vi "Lab Panel V4.90.vi"() -> ()   [LabVIEW 2013] (continued)
                    n2521 = local read "SIG LAB02-2"() -> (w4767:T2)
                    n2522 = local read "RESULT LAB02-2"() -> (w4754:bool)
                    n2523 = Bundle("FAIL LAB02-2"=w4757, "SIG LAB02-2"=w4767, "TEMP START LAB02-2"=w4766, "DISP LAB02-2"=w4763, "SET LAB02-2"=w4762, "TDMS LAB02-2"=w4765) -> (w4752:T35)  [unwired: 1 in]
                    n2524 = call "sub vi - cycle&temp fail v7.vi"("Amps Lo?"=w4764, "Input Cluster"=w4752, "SELECT"=w4761, "Amps Hi?"=w4760, "Result In"=w4754) -> ("(FAIL) out"=w4756:cluster{"FAIL LO":dbl, "FAIL HI":dbl}, "(DISP) out"=w4759:T4, "T-RISE"=w4753:cluster{"T-RISE (L)":dbl, "T-RISE (N)":dbl}, "Result Out"=w4755:bool, "file error"=w4758:errorcluster)  [unwired: 10 in]
                    n2525 = local write "TEMP RISE LAB02-2"(w4753) -> ()
                    n2526 = local write "FAIL LAB02-2"(w4756) -> ()
                    n2527 = local write "DISP LAB02-2"(w4759) -> ()
                    n2528 = local write "RESULT LAB02-2"(w4755) -> ()
                    n2529 = local write "data file error"(w4758) -> ()
                  }
                }
              }
              frame #4 {
                # "LAB03-1"
                n2530 = case shown="True" w4769 {
                  tunnel: w4771 -> [_ w4784]
                  tunnel: w4768 -> [_ w4781]
                  tunnel: w4770 -> [_ w4780]
                  frame False {
                  }
                  frame True {
                    n2531 = local read "TEMP START LAB03-1"() -> (w4786:cluster{"TL":dbl, "TN":dbl})
                    n2532 = local read "FAIL LAB03-1"() -> (w4777:cluster{"LO":dbl, "HI":dbl})
                    n2533 = local read "TDMS LAB03-1"() -> (w4785:refnum<k34>)
                    n2534 = local read "SET LAB03-1"() -> (w4782:T5)
                    n2535 = local read "DISP LAB03-1"() -> (w4783:T4)
                    n2536 = local read "SIG LAB03-1"() -> (w4787:T2)
                    n2537 = local read "RESULT LAB03-1"() -> (w4774:bool)
                    n2538 = Bundle("FAIL LAB03-1"=w4777, "SIG LAB03-1"=w4787, "TEMP START LAB03-1"=w4786, "DISP LAB03-1"=w4783, "SET LAB03-1"=w4782, "TDMS LAB03-1"=w4785) -> (w4772:T36)  [unwired: 1 in]
                    n2539 = call "sub vi - cycle&temp fail v7.vi"("Amps Lo?"=w4784, "Input Cluster"=w4772, "SELECT"=w4781, "Amps Hi?"=w4780, "Result In"=w4774) -> ("(FAIL) out"=w4776:cluster{"FAIL LO":dbl, "FAIL HI":dbl}, "(DISP) out"=w4779:T4, "T-RISE"=w4773:cluster{"T-RISE (L)":dbl, "T-RISE (N)":dbl}, "Result Out"=w4775:bool, "file error"=w4778:errorcluster)  [unwired: 10 in]
                    n2540 = local write "TEMP RISE LAB03-1"(w4773) -> ()
                    n2541 = local write "FAIL LAB03-1"(w4776) -> ()
                    n2542 = local write "DISP LAB03-1"(w4779) -> ()
                    n2543 = local write "RESULT LAB03-1"(w4775) -> ()
                    n2544 = local write "data file error"(w4778) -> ()
                  }
                }
              }
              frame #5 {
                # "LAB03-2"
                n2545 = case shown="True" w4789 {
                  tunnel: w4791 -> [_ w4804]
                  tunnel: w4788 -> [_ w4801]
                  tunnel: w4790 -> [_ w4800]
                  frame False {
                  }
                  frame True {
                    n2546 = local read "TEMP START LAB03-2"() -> (w4806:cluster{"TL":dbl, "TN":dbl})
                    n2547 = local read "FAIL LAB03-2"() -> (w4797:cluster{"LO":dbl, "HI":dbl})
                    n2548 = local read "TDMS LAB03-2"() -> (w4805:refnum<k34>)
                    n2549 = local read "SET LAB03-2"() -> (w4802:T5)
                    n2550 = local read "DISP LAB03-2"() -> (w4803:T4)
                    n2551 = local read "RESULT LAB03-2"() -> (w4794:bool)
                    n2552 = local read "SIG LAB03-2"() -> (w4807:T2)
                    n2553 = Bundle("FAIL LAB03-2"=w4797, "SIG LAB03-2"=w4807, "TEMP START LAB03-2"=w4806, "DISP LAB03-2"=w4803, "SET LAB03-2"=w4802, "TDMS LAB03-2"=w4805) -> (w4792:T37)  [unwired: 1 in]
                    n2554 = call "sub vi - cycle&temp fail v7.vi"("Amps Lo?"=w4804, "Input Cluster"=w4792, "SELECT"=w4801, "Amps Hi?"=w4800, "Result In"=w4794) -> ("(FAIL) out"=w4796:cluster{"FAIL LO":dbl, "FAIL HI":dbl}, "(DISP) out"=w4799:T4, "T-RISE"=w4793:cluster{"T-RISE (L)":dbl, "T-RISE (N)":dbl}, "Result Out"=w4795:bool, "file error"=w4798:errorcluster)  [unwired: 10 in]
                    n2555 = local write "FAIL LAB03-2"(w4796) -> ()
                    n2556 = local write "TEMP RISE LAB03-2"(w4793) -> ()
                    n2557 = local write "DISP LAB03-2"(w4799) -> ()
                    n2558 = local write "RESULT LAB03-2"(w4795) -> ()
                    n2559 = local write "data file error"(w4798) -> ()
                  }
                }
              }
              frame #6 {
                # "LAB04-1"
                n2560 = case shown="True" w4809 {
                  tunnel: w4811 -> [_ w4824]
                  tunnel: w4808 -> [_ w4821]
                  tunnel: w4810 -> [_ w4820]
                  frame False {
                  }
                  frame True {
                    n2561 = local read "TEMP START LAB04-1"() -> (w4826:cluster{"TL":dbl, "TN":dbl})
                    n2562 = local read "FAIL LAB04-1"() -> (w4817:cluster{"LO":dbl, "HI":dbl})
                    n2563 = local read "TDMS LAB04-1"() -> (w4825:refnum<k34>)
                    n2564 = local read "SET LAB04-1"() -> (w4822:T5)
                    n2565 = local read "DISP LAB04-1"() -> (w4823:T4)
                    n2566 = local read "SIG LAB04-1"() -> (w4827:T2)
                    n2567 = local read "RESULT LAB04-1"() -> (w4814:bool)
                    n2568 = Bundle("FAIL LAB04-1"=w4817, "SIG LAB04-1"=w4827, "TEMP START LAB04-1"=w4826, "DISP LAB04-1"=w4823, "SET LAB04-1"=w4822, "TDMS LAB04-1"=w4825) -> (w4812:T38)  [unwired: 1 in]
                    n2569 = call "sub vi - cycle&temp fail v7.vi"("Amps Lo?"=w4824, "Input Cluster"=w4812, "SELECT"=w4821, "Amps Hi?"=w4820, "Result In"=w4814) -> ("(FAIL) out"=w4816:cluster{"FAIL LO":dbl, "FAIL HI":dbl}, "(DISP) out"=w4819:T4, "T-RISE"=w4813:cluster{"T-RISE (L)":dbl, "T-RISE (N)":dbl}, "Result Out"=w4815:bool, "file error"=w4818:errorcluster)  [unwired: 10 in]
                    n2570 = local write "TEMP RISE LAB04-1"(w4813) -> ()
                    n2571 = local write "FAIL LAB04-1"(w4816) -> ()
                    n2572 = local write "DISP LAB04-1"(w4819) -> ()
                    n2573 = local write "RESULT LAB04-1"(w4815) -> ()
                    n2574 = local write "data file error"(w4818) -> ()
                  }
                }
              }
              frame #7 {
                # "LAB04-2"
                n2575 = case shown="True" w4829 {
                  tunnel: w4831 -> [_ w4844]
                  tunnel: w4828 -> [_ w4841]
                  tunnel: w4830 -> [_ w4840]
                  frame False {
                  }
                  frame True {
                    n2576 = local read "TEMP START LAB04-2"() -> (w4846:cluster{"TL":dbl, "TN":dbl})
                    n2577 = local read "FAIL LAB04-2"() -> (w4837:cluster{"LO":dbl, "HI":dbl})
                    n2578 = local read "TDMS LAB04-2"() -> (w4845:refnum<k34>)
                    n2579 = local read "SET LAB04-2"() -> (w4842:T5)
                    n2580 = local read "DISP LAB04-2"() -> (w4843:T4)
                    n2581 = local read "SIG LAB04-2"() -> (w4847:T2)
                    n2582 = local read "RESULT LAB04-2"() -> (w4834:bool)
                    n2583 = Bundle("FAIL LAB04-2"=w4837, "SIG LAB04-2"=w4847, "TEMP START LAB04-2"=w4846, "DISP LAB04-2"=w4843, "SET LAB04-2"=w4842, "TDMS LAB04-2"=w4845) -> (w4832:T39)  [unwired: 1 in]
                    n2584 = call "sub vi - cycle&temp fail v7.vi"("Amps Lo?"=w4844, "Input Cluster"=w4832, "SELECT"=w4841, "Amps Hi?"=w4840, "Result In"=w4834) -> ("(FAIL) out"=w4836:cluster{"FAIL LO":dbl, "FAIL HI":dbl}, "(DISP) out"=w4839:T4, "T-RISE"=w4833:cluster{"T-RISE (L)":dbl, "T-RISE (N)":dbl}, "Result Out"=w4835:bool, "file error"=w4838:errorcluster)  [unwired: 10 in]
                    n2585 = local write "TEMP RISE LAB04-2"(w4833) -> ()
                    n2586 = local write "FAIL LAB04-2"(w4836) -> ()
                    n2587 = local write "DISP LAB04-2"(w4839) -> ()
                    n2588 = local write "RESULT LAB04-2"(w4835) -> ()
                    n2589 = local write "data file error"(w4838) -> ()
                  }
                }
              }
              frame #8 {
                # "LAB05-1"
                n2590 = case shown="True" w4849 {
                  tunnel: w4851 -> [_ w4864]
                  tunnel: w4848 -> [_ w4861]
                  tunnel: w4850 -> [_ w4860]
                  frame False {
                  }
                  frame True {
                    n2591 = local read "TEMP START LAB05-1"() -> (w4866:cluster{"TL":dbl, "TN":dbl})
                    n2592 = local read "FAIL LAB05-1"() -> (w4857:cluster{"LO":dbl, "HI":dbl})
                    n2593 = local read "TDMS LAB05-1"() -> (w4865:refnum<k34>)
                    n2594 = local read "SET LAB05-1"() -> (w4862:T5)
                    n2595 = local read "DISP LAB05-1"() -> (w4863:T4)
                    n2596 = local read "SIG LAB05-1"() -> (w4867:T2)
                    n2597 = local read "RESULT LAB05-1"() -> (w4854:bool)
                    n2598 = Bundle("FAIL LAB05-1"=w4857, "SIG LAB05-1"=w4867, "TEMP START LAB05-1"=w4866, "DISP LAB05-1"=w4863, "SET LAB05-1"=w4862, "TDMS LAB05-1"=w4865) -> (w4852:T40)  [unwired: 1 in]
                    n2599 = call "sub vi - cycle&temp fail v7.vi"("Amps Lo?"=w4864, "Input Cluster"=w4852, "SELECT"=w4861, "Amps Hi?"=w4860, "Result In"=w4854) -> ("(FAIL) out"=w4856:cluster{"FAIL LO":dbl, "FAIL HI":dbl}, "(DISP) out"=w4859:T4, "T-RISE"=w4853:cluster{"T-RISE (L)":dbl, "T-RISE (N)":dbl}, "Result Out"=w4855:bool, "file error"=w4858:errorcluster)  [unwired: 10 in]
                    n2600 = local write "TEMP RISE LAB05-1"(w4853) -> ()
                    n2601 = local write "FAIL LAB05-1"(w4856) -> ()
                    n2602 = local write "DISP LAB05-1"(w4859) -> ()
                    n2603 = local write "RESULT LAB05-1"(w4855) -> ()
                    n2604 = local write "data file error"(w4858) -> ()
                  }
                }
              }
              frame #9 {
                # "LAB05-2"
                n2605 = case shown="True" w4869 {
                  tunnel: w4871 -> [_ w4884]
                  tunnel: w4868 -> [_ w4881]
                  tunnel: w4870 -> [_ w4880]
                  frame False {
                  }
                  frame True {
                    n2606 = local read "TEMP START LAB05-2"() -> (w4886:cluster{"TL":dbl, "TN":dbl})
                    n2607 = local read "FAIL LAB05-2"() -> (w4877:cluster{"LO":dbl, "HI":dbl})
                    n2608 = local read "TDMS LAB05-2"() -> (w4885:refnum<k34>)
                    n2609 = local read "SET LAB05-2"() -> (w4882:T5)
                    n2610 = local read "DISP LAB05-2"() -> (w4883:T4)
                    n2611 = local read "SIG LAB05-2"() -> (w4887:T2)
                    n2612 = local read "RESULT LAB05-2"() -> (w4874:bool)
                    n2613 = Bundle("FAIL LAB05-2"=w4877, "SIG LAB05-2"=w4887, "TEMP START LAB05-2"=w4886, "DISP LAB05-2"=w4883, "SET LAB05-2"=w4882, "TDMS LAB05-2"=w4885) -> (w4872:T41)  [unwired: 1 in]
                    n2614 = call "sub vi - cycle&temp fail v7.vi"("Amps Lo?"=w4884, "Input Cluster"=w4872, "SELECT"=w4881, "Amps Hi?"=w4880, "Result In"=w4874) -> ("(FAIL) out"=w4876:cluster{"FAIL LO":dbl, "FAIL HI":dbl}, "(DISP) out"=w4879:T4, "T-RISE"=w4873:cluster{"T-RISE (L)":dbl, "T-RISE (N)":dbl}, "Result Out"=w4875:bool, "file error"=w4878:errorcluster)  [unwired: 10 in]
                    n2615 = local write "TEMP RISE LAB05-2"(w4873) -> ()
                    n2616 = local write "FAIL LAB05-2"(w4876) -> ()
                    n2617 = local write "DISP LAB05-2"(w4879) -> ()
                    n2618 = local write "RESULT LAB05-2"(w4875) -> ()
                    n2619 = local write "data file error"(w4878) -> ()
                  }
                }
              }
            }
          }
          frame #15 {
            # "run calibration routine"
            n2620 = local read "SET (cal)"() -> (w4888:bool)
            n2621 = case shown="True" w4888 {
              frame False {
              }
              frame True {
                n2622 = stacked-sequence {
                  seq-local: [w4889 _ _] -> [_ w4891 _]
                  frame #0 {
                    n2623 = call "CALIBRATION PASSWORD"() -> ("PASSWORD"=w4889:string)  [unwired: 17 in, 2 out]
                  }
                  frame #1 {
                    n2624 = Equal?(x=w4891, y="7777") -> (x = y?=w4890:bool)
                    n2625 = case shown="True" w4890 {
                      frame False {
                      }
                      frame True {
                        n2626 = stacked-sequence {
                          frame #0 {
                            n2627 = local read "Temp Test Cal"() -> (w4893:dbl)
                            n2628 = call "sub vi - calibration v1.vi"("Temp Test Cal"=w4893) -> ()  [unwired: 11 in]
                          }
                          frame #1 {
                            n2629 = call "sub vi - get calibration values v1.vi"() -> ("TEMP REF CAL"=w4894:dbl, "LAB01 (CAL)"=w4899:T14, "LAB02 (CAL)"=w4898:T15, "LAB03 (CAL)"=w4897:T14, "LAB04 (CAL)"=w4896:T14, "calibration file error out"=w4900:errorcluster, "LAB05 (CAL)"=w4895:T14)  [unwired: 9 in]
                            n2630 = local write "TEMP REF cal"(w4894) -> ()
                            n2631 = local write "cal file error out"(w4900) -> ()
                            n2632 = local write "CAL LAB04"(w4896) -> ()
                            n2633 = local write "CAL LAB05"(w4895) -> ()
                            n2634 = local write "CAL LAB01"(w4899) -> ()
                            n2635 = local write "CAL LAB02"(w4898) -> ()
                            n2636 = local write "CAL LAB03"(w4897) -> ()
                          }
                        }
                      }
                    }
                  }
                  frame #2 {
                    n2637 = local write "SET (cal)"(FALSE) -> ()
                  }
                }
              }
            }
          }
          frame #16 {
            # "save certain settings to file"
            n2638 = String To Path(string="c:\\crabtree\\Set Up\\") -> (path=w4903:path)
            n2639 = Build Path(base path=w4903, name or relative path="settings.bin") -> (appended path=w4905:path)
            n2640 = Build Path(base path=w4903, name or relative path="mail.bin") -> (appended path=w4902:path)
            n2641 = Create Folder(path (use dialog)=w4903) -> (error out=w4908:errorcluster)  [unwired: 2 in, 2 out]
            n2642 = call <vilib>:"Clear Errors.vi"("error in (no error)"=w4908) -> ()  [unwired: 6 in, 1 out]
            n2643 = stacked-sequence {
              seq-local: [w4920 _] -> [_ w4933]
              tunnel: w4905 -> [_ w4934]
              tunnel: w4902 -> [_ w4932]
              frame #0 {
                n2644 = local read "C drive data root dir"() -> (w4919:path)
                n2645 = local read "Select COM port"() -> (w4916:refnum<visa-resource-name>)
                n2646 = local read "Network Directory"() -> (w4925:path)
                n2647 = local read "SET LAB05-2"() -> (w4924:T5)
                n2648 = local read "SET LAB05-1"() -> (w4923:T5)
                n2649 = local read "SET LAB04-2"() -> (w4922:T5)
                n2650 = local read "SET LAB03-2"() -> (w4926:T5)
                n2651 = local read "SET LAB04-1"() -> (w4921:T5)
                n2652 = local read "SET LAB03-1"() -> (w4927:T5)
                n2653 = local read "SET LAB02-2"() -> (w4928:T5)
                n2654 = local read "SET LAB02-1"() -> (w4929:T5)
                n2655 = local read "Temp Delay Lps"() -> (w4915:dbl)
                n2656 = local read "Amps Fail level"() -> (w4911:dbl)
                n2657 = local read "SET LAB01-2"() -> (w4930:T5)
                n2658 = local read "Temp Test Cal"() -> (w4912:dbl)
                n2659 = local read "SET LAB01-1"() -> (w4931:T5)
                n2660 = local read "Mail Test File To:"() -> (w4910:string)
                n2661 = local read "Temp Value"() -> (w4914:dbl)
                n2662 = local read "Fail Loops"() -> (w4913:dbl)
                n2663 = local read "Mail Test Fail"() -> (w4909:bool)
                n2664 = local read "RATE (Hz)"() -> (w4918:dbl)
                n2665 = local read "SAMPLES"() -> (w4917:dbl)
                n2666 = Bundle("SET LAB01-1"=w4931, "SET LAB01-2"=w4930, "SET LAB02-1"=w4929, "SET LAB02-2"=w4928, "SET LAB03-1"=w4927, "SET LAB03-2"=w4926, "SET LAB04-1"=w4921, "SET LAB04-2"=w4922, "SET LAB05-1"=w4923, "SET LAB05-2"=w4924, "Network Directory"=w4925, "C drive data root dir"=w4919, "RATE (Hz)"=w4918, "SAMPLES"=w4917, "Select COM port"=w4916, "Temp Delay Lps"=w4915, "Temp Value"=w4914, "Fail Loops"=w4913, "Temp Test Cal"=w4912, "Amps Fail level"=w4911, "Mail Test File To:"=w4910, "Mail Test Fail"=w4909) -> (w4920:T22)  [unwired: 1 in]
              }
              frame #1 {
                n2667 = event shown="[1] \"SET LAB01-1\", \"SET LAB01-2\", \"SET LAB02-1\", \"SET LAB02-2\", \"SET LAB03-1\", \"SET LAB03-2\", \"SET LAB04-1\", \"SET LAB04-2\", \"SET LAB05-1\", \"SET LAB05-2\", \"Network Directory\", \"C drive data root dir\", \"RATE (Hz)\", \"SAMPLES\", \"Select COM port\", \"Temp Delay Lps\", \"Temp Value\", \"Fail Loops\", \"Temp Test Cal\", \"Amps Fail level\", \"Mail Test File To:\", \"Mail Test Fail\": Value Change" {
                  selector: _ -> [_ _ _]
                  dyn-events: _ -> [_ _ _]
                  timeout: 10.0 -> [_ _ _]
                  tunnel: w4934 -> [_ w4936 _]
                  tunnel: w4933 -> [_ w4937 _]
                  tunnel: w4932 -> [_ _ w4948]
                  event Timeout {
                    n2668 = event-data() -> ()  [unwired: 1 in, 3 out]
                  }
                  event "SET LAB01-1", "SET LAB01-2", "SET LAB02-1", "SET LAB02-2", "SET LAB03-1", "SET LAB03-2", "SET LAB04-1", "SET LAB04-2", "SET LAB05-1", "SET LAB05-2", "Network Directory", "C drive data root dir", "RATE (Hz)", "SAMPLES", "Select COM port", "Temp Delay Lps", "Temp Value", "Fail Loops", "Temp Test Cal", "Amps Fail level", "Mail Test File To:", "Mail Test Fail": Value Change {
                    n2669 = event-data() -> ()  [unwired: 1 in, 6 out]
                    n2670 = Open/Create/Replace File(file path (use dialog)=w4936, operation (0:open)=T21."replace or create") -> (refnum out=w4942:refnum<file>, error out=w4941:errorcluster)  [unwired: 4 in, 1 out]
                    n2671 = Write to Binary File(file (use dialog)=w4942, data=w4937, error in=w4941) -> (refnum out=w4940:refnum<file>, error out=w4939:errorcluster)  [unwired: 3 in, 1 out]
                    n2672 = Close File(refnum=w4940, error in=w4939) -> (error out=w4938:errorcluster)  [unwired: 1 out]
                    n2673 = local write "data file error"(w4938) -> ()
                  }
                  event "MAIL SETTINGS.OUT SERVER ADDRESS", "MAIL SETTINGS.FROM ACCOUNT", "MAIL SETTINGS.USER NAME", "MAIL SETTINGS.PASSWORD", "Auto Mail Send", "TO (string):": Value Change {
                    n2674 = event-data() -> ()  [unwired: 1 in, 6 out]
                    n2675 = local read "MAIL SETTINGS"() -> (w4947:T7)
                    n2676 = local read "Auto Mail Send"() -> (w4945:bool)
                    n2677 = local read "TO (string):"() -> (w4944:string)
                    n2678 = Open/Create/Replace File(file path (use dialog)=w4948, operation (0:open)=T21."replace or create") -> (refnum out=w4953:refnum<file>, error out=w4952:errorcluster)  [unwired: 4 in, 1 out]
                    n2679 = Bundle("MAIL SETTINGS"=w4947, "Auto Mail Send"=w4945, "TO (string):"=w4944) -> (w4946:T42)  [unwired: 1 in]
                    n2680 = Write to Binary File(file (use dialog)=w4953, data=w4946, error in=w4952) -> (refnum out=w4951:refnum<file>, error out=w4950:errorcluster)  [unwired: 3 in, 1 out]
                    n2681 = Close File(refnum=w4951, error in=w4950) -> (error out=w4949:errorcluster)  [unwired: 1 out]
                    n2682 = local write "data file error"(w4949) -> ()
                  }
                }
              }
            }
          }
          frame #17 {
            # "mail control"
            n2683 = local read "MAIL SETTINGS"() -> (w4970:T7)
            n2684 = local read "Auto Mail Send"() -> (w4956:bool)
            n2685 = Unbundle(w4970) -> ("OUT SERVER ADDRESS"=w4969:string, "FROM ACCOUNT"=w4968:string, "TEST MAIL"=w4967:bool)  [unwired: 4 out]
            n2686 = stacked-sequence {
              tunnel: "TO (string):" -> [_ w5009]
              tunnel: w4970 -> [w4975 w5008]
              tunnel: w4969 -> [w4974 w5007]
              tunnel: w4968 -> [w4973 w5006]
              tunnel: w4967 -> [w4972 _]
              tunnel: w4956 -> [_ w5005]
              tunnel: w4966 -> [_ w5004]
              tunnel: w4965 -> [_ w5003]
              tunnel: w4964 -> [_ w5002]
              tunnel: w4963 -> [_ w5001]
              tunnel: w4962 -> [_ w5000]
              tunnel: w4961 -> [_ w4999]
              tunnel: w4960 -> [_ w4998]
              tunnel: w4959 -> [_ w4997]
              tunnel: w4958 -> [_ w4996]
              tunnel: w4957 -> [_ w4995]
              tunnel: "TO (string):" -> [w4971 _]
              frame #0 {
                # "mail test"
                n2687 = case shown="True" w4972 {
                  tunnel: w4975 -> [_ w4979]
                  tunnel: w4971 -> [_ w4978]
                  tunnel: w4974 -> [_ w4977]
                  tunnel: w4973 -> [_ w4976]
                  frame False {
                  }
                  frame True {
                    n2688 = stacked-sequence {
                      seq-local: [_ _ w4989 _] -> [_ _ _ w4990]
                      tunnel: w4979 -> [w4982 _ _ w4994]
                      tunnel: w4978 -> [_ _ w4987 _]
                      tunnel: w4977 -> [_ _ w4985 _]
                      tunnel: w4976 -> [_ _ w4986 _]
                      frame #0 {
                        n2689 = Bundle(cluster=w4982, "TEST MAIL STATUS"="TEST START") -> (w4980:T7)  [unwired: 6 in]
                        n2690 = local write "MAIL SETTINGS"(w4980) -> ()
                      }
                      frame #1 {
                        n2691 = Wait (ms)(milliseconds to wait=500) -> ()  [unwired: 1 out]
                      }
                      frame #2 {
                        n2692 = call "sub vi - send mail v5.vi"("TO:"=w4987, "subject"="MAIL TEST FROM LAB PANEL", "from"=w4986, "out going server"=w4985, "message"="TEST MESSAGE") -> ("error out"=w4989:errorcluster)  [unwired: 10 in]
                      }
                      frame #3 {
                        n2693 = Bundle(cluster=w4994, "TEST MAIL"=FALSE, "TEST MAIL STATUS"="TEST END", "mail error"=w4990) -> (w4992:T7)  [unwired: 4 in]
                        n2694 = local write "MAIL SETTINGS"(w4992) -> ()
                      }
                    }
                  }
                }
              }
              frame #1 {
                # "mail report"
                n2695 = stacked-sequence {
                  seq-local: [_ w5052 _ _] -> [_ _ _ w5242]
                  seq-local: [_ _ w5155 _] -> [_ _ _ w5232]
                  seq-local: [w5019 _ _ _] -> [_ w5069 _ _]
                  seq-local: [w5018 _ _ _] -> [_ w5068 _ _]
                  seq-local: [w5016 _ _ _] -> [_ w5066 _ _]
                  seq-local: [w5017 _ _ _] -> [_ w5067 _ _]
                  seq-local: [w5015 _ _ _] -> [_ w5065 _ _]
                  seq-local: [w5014 _ _ _] -> [_ w5060 _ _]
                  seq-local: [w5013 _ _ _] -> [_ w5061 _ _]
                  seq-local: [w5012 _ _ _] -> [_ w5062 _ _]
                  seq-local: [w5011 _ _ _] -> [_ w5063 _ _]
                  seq-local: [w5010 _ _ _] -> [_ w5064 _ _]
                  tunnel: w5009 -> [_ _ _ w5243]
                  tunnel: w5008 -> [_ _ _ w5226]
                  tunnel: w5007 -> [_ _ _ w5240]
                  tunnel: w5006 -> [_ _ _ w5239]
                  tunnel: w5005 -> [w5050 _ _ w5234]
                  tunnel: w5004 -> [_ _ w5185 _]
                  tunnel: w5003 -> [_ _ w5182 _]
                  tunnel: w5002 -> [_ _ w5181 _]
                  tunnel: w5001 -> [_ _ w5180 _]
                  tunnel: w5000 -> [_ _ w5179 _]
                  tunnel: w4999 -> [_ _ w5178 _]
                  tunnel: w4998 -> [_ _ w5177 _]
                  tunnel: w4997 -> [_ _ w5176 _]
                  tunnel: w4996 -> [_ _ w5175 _]
                  tunnel: w4995 -> [_ _ w5174 _]
                  frame #0 {
                    n2696 = case shown="False" w5050 {
                      frame False {
                        n2697 = local write "mail control"("") -> ()
                      }
                      frame True {
                      }
                    }
                    n2698 = local read "SET LAB01-1"() -> (w5049:T5)
                    n2699 = local read "SET LAB01-2"() -> (w5048:T5)
                    n2700 = local read "SET LAB02-1"() -> (w5047:T5)
                    n2701 = local read "SET LAB02-2"() -> (w5046:T5)
                    n2702 = local read "SET LAB03-1"() -> (w5045:T5)
                    n2703 = local read "SET LAB04-1"() -> (w5043:T5)
                    n2704 = local read "SET LAB05-1"() -> (w5041:T5)
                    n2705 = local read "SET LAB03-2"() -> (w5044:T5)
                    n2706 = local read "SET LAB04-2"() -> (w5042:T5)
                    n2707 = local read "SET LAB05-2"() -> (w5040:T5)
                    n2708 = Unbundle(w5045) -> ("DESCRIPTION"=w5025:string)  [unwired: 4 out]
                    n2709 = Unbundle(w5044) -> ("DESCRIPTION"=w5024:string)  [unwired: 4 out]
                    n2710 = Unbundle(w5043) -> ("DESCRIPTION"=w5023:string)  [unwired: 4 out]
                    n2711 = Unbundle(w5040) -> ("DESCRIPTION"=w5020:string)  [unwired: 4 out]
                    n2712 = Unbundle(w5046) -> ("DESCRIPTION"=w5026:string)  [unwired: 4 out]
                    n2713 = Unbundle(w5042) -> ("DESCRIPTION"=w5022:string)  [unwired: 4 out]
                    n2714 = Unbundle(w5049) -> ("DESCRIPTION"=w5038:string)  [unwired: 4 out]
                    n2715 = Unbundle(w5047) -> ("DESCRIPTION"=w5027:string)  [unwired: 4 out]
                    n2716 = Unbundle(w5041) -> ("DESCRIPTION"=w5021:string)  [unwired: 4 out]
                    n2717 = Unbundle(w5048) -> ("DESCRIPTION"=w5028:string)  [unwired: 4 out]
                    n2718 = Concatenate Strings("[LAB05-2/", w5020) -> (w5010:string)
                    n2719 = Concatenate Strings("[LAB05-1/", w5021) -> (w5011:string)
                    n2720 = Concatenate Strings("[LAB04-2/", w5022) -> (w5012:string)
                    n2721 = Concatenate Strings("[LAB03-2/", w5024) -> (w5014:string)
                    n2722 = Concatenate Strings("[LAB04-1/", w5023) -> (w5013:string)
                    n2723 = Concatenate Strings("[LAB03-1/", w5025) -> (w5015:string)
                    n2724 = Concatenate Strings("[LAB01-2/", w5028) -> (w5018:string)
                    n2725 = Concatenate Strings("[LAB02-2/", w5026) -> (w5016:string)
                    n2726 = Concatenate Strings("[LAB01-1/", w5038) -> (w5019:string)
                    n2727 = Concatenate Strings("[LAB02-1/", w5027) -> (w5017:string)
                  }
                  frame #1 {
                    w5073 = "/"
                    w5074 = 2.0
                    n2728 = local read "DISP LAB01-2"() -> (w5153:T4)
                    n2729 = local read "DISP LAB01-1"() -> (w5154:T4)
                    n2730 = local read "DISP LAB02-1"() -> (w5152:T4)
                    n2731 = local read "DISP LAB03-2"() -> (w5149:T4)
                    n2732 = local read "DISP LAB02-2"() -> (w5151:T4)
                    n2733 = local read "DISP LAB03-1"() -> (w5150:T4)
                    n2734 = local read "DISP LAB04-2"() -> (w5147:T4)
                    n2735 = local read "DISP LAB04-1"() -> (w5148:T4)
                    n2736 = local read "DISP LAB05-1"() -> (w5146:T4)
                    n2737 = local read "DISP LAB05-2"() -> (w5145:T4)
                    n2738 = Unbundle(w5153) -> ("CYCLE"=w5137:dbl, "MINS"=w5136:dbl, "STATUS"=w5133:string)
                    n2739 = Unbundle(w5154) -> ("CYCLE"=w5142:dbl, "MINS"=w5141:dbl, "STATUS"=w5138:string)
                    n2740 = Unbundle(w5152) -> ("CYCLE"=w5130:dbl, "MINS"=w5129:dbl, "STATUS"=w5128:string)
                    n2741 = Unbundle(w5149) -> ("CYCLE"=w5117:dbl, "MINS"=w5116:dbl, "STATUS"=w5113:string)
                    n2742 = Unbundle(w5150) -> ("CYCLE"=w5122:dbl, "MINS"=w5121:dbl, "STATUS"=w5118:string)
                    n2743 = Unbundle(w5151) -> ("CYCLE"=w5127:dbl, "MINS"=w5126:dbl, "STATUS"=w5123:string)
                    n2744 = Unbundle(w5148) -> ("CYCLE"=w5112:dbl, "MINS"=w5111:dbl, "STATUS"=w5108:string)
                    n2745 = Unbundle(w5147) -> ("CYCLE"=w5107:dbl, "MINS"=w5106:dbl, "STATUS"=w5103:string)
                    n2746 = Unbundle(w5146) -> ("CYCLE"=w5102:dbl, "MINS"=w5101:dbl, "STATUS"=w5098:string)
                    n2747 = Unbundle(w5145) -> ("CYCLE"=w5144:dbl, "MINS"=w5143:dbl, "STATUS"=w5095:string)
                    n2748 = Number To Decimal String(number=w5130) -> (decimal integer string=w5132:string)  [unwired: 1 in]
                    n2749 = Number To Decimal String(number=w5127) -> (decimal integer string=w5125:string)  [unwired: 1 in]
                    n2750 = Number To Decimal String(number=w5122) -> (decimal integer string=w5120:string)  [unwired: 1 in]
                    n2751 = Number To Decimal String(number=w5137) -> (decimal integer string=w5135:string)  [unwired: 1 in]
                    n2752 = Number To Decimal String(number=w5117) -> (decimal integer string=w5115:string)  [unwired: 1 in]
                    n2753 = Number To Decimal String(number=w5142) -> (decimal integer string=w5140:string)  [unwired: 1 in]
                    n2754 = Number To Decimal String(number=w5144) -> (decimal integer string=w5097:string)  [unwired: 1 in]
                    n2755 = Number To Decimal String(number=w5112) -> (decimal integer string=w5110:string)  [unwired: 1 in]
                    n2756 = Number To Decimal String(number=w5107) -> (decimal integer string=w5105:string)  [unwired: 1 in]
                    n2757 = Number To Decimal String(number=w5102) -> (decimal integer string=w5100:string)  [unwired: 1 in]
                    n2758 = Number To Fractional String(number=w5129, precision (6)=w5074) -> (F-format string=w5131:string)  [unwired: 2 in]
                    n2759 = Number To Fractional String(number=w5116, precision (6)=w5074) -> (F-format string=w5114:string)  [unwired: 2 in]
                    n2760 = Number To Fractional String(number=w5126, precision (6)=w5074) -> (F-format string=w5124:string)  [unwired: 2 in]
                    n2761 = Number To Fractional String(number=w5121, precision (6)=w5074) -> (F-format string=w5119:string)  [unwired: 2 in]
                    n2762 = Number To Fractional String(number=w5106, precision (6)=w5074) -> (F-format string=w5104:string)  [unwired: 2 in]
                    n2763 = Number To Fractional String(number=w5111, precision (6)=w5074) -> (F-format string=w5109:string)  [unwired: 2 in]
                    n2764 = Number To Fractional String(number=w5136, precision (6)=w5074) -> (F-format string=w5134:string)  [unwired: 2 in]
                    n2765 = Number To Fractional String(number=w5101, precision (6)=w5074) -> (F-format string=w5099:string)  [unwired: 2 in]
                    n2766 = Number To Fractional String(number=w5141, precision (6)=w5074) -> (F-format string=w5139:string)  [unwired: 2 in]
                    n2767 = Number To Fractional String(number=w5143, precision (6)=w5074) -> (F-format string=w5096:string)  [unwired: 2 in]
                    n2768 = Concatenate Strings(w5073, w5115, w5073, w5114, w5073, w5113) -> (w5089:string)
                    n2769 = Concatenate Strings(w5073, w5110, w5073, w5109, w5073, w5108) -> (w5088:string)
                    n2770 = Concatenate Strings(w5073, w5105, w5073, w5104, w5073, w5103) -> (w5087:string)
                    n2771 = Concatenate Strings(w5073, w5100, w5073, w5099, w5073, w5098) -> (w5086:string)
                    n2772 = Concatenate Strings(w5073, w5097, w5073, w5096, w5073, w5095) -> (w5085:string)
                    n2773 = Concatenate Strings(w5073, w5140, w5073, w5139, w5073, w5138) -> (w5094:string)
                    n2774 = Concatenate Strings(w5073, w5120, w5073, w5119, w5073, w5118) -> (w5090:string)
                    n2775 = Concatenate Strings(w5073, w5135, w5073, w5134, w5073, w5133) -> (w5093:string)
                    n2776 = Concatenate Strings(w5073, w5132, w5073, w5131, w5073, w5128) -> (w5092:string)
                    n2777 = Concatenate Strings(w5073, w5125, w5073, w5124, w5073, w5123) -> (w5091:string)
                    n2778 = Concatenate Strings("]", "\r") -> (w5070:string)
                    n2779 = Concatenate Strings(w5065, w5090, w5070) -> (w5080:string)
                    n2780 = Concatenate Strings(w5067, w5092, w5070) -> (w5082:string)
                    n2781 = Concatenate Strings(w5066, w5091, w5070) -> (w5081:string)
                    n2782 = Concatenate Strings(w5062, w5087, w5070) -> (w5077:string)
                    n2783 = Concatenate Strings(w5063, w5086, w5070) -> (w5078:string)
                    n2784 = Concatenate Strings(w5061, w5088, w5070) -> (w5076:string)
                    n2785 = Concatenate Strings(w5060, w5089, w5070) -> (w5075:string)
                    n2786 = Concatenate Strings(w5064, w5085, w5070) -> (w5079:string)
                    n2787 = Concatenate Strings(w5068, w5093, w5070) -> (w5083:string)
                    n2788 = Concatenate Strings(w5069, w5094, w5070) -> (w5084:string)
                    n2789 = Concatenate Strings(w5084, w5083, w5082, w5081, w5080, w5075, w5076, w5077, w5078, w5079) -> (w5053:string)
                    n2790 = Concatenate Strings("[PANEL/", "DESC/", "CYCLES/", "MINS/", "STATUS]", "\r", w5053) -> (w5052:string)
                    "MAIL REPORT" <- w5052
                    n2791 = global write "Global display 3.vi" "log all"(w5052) -> ()
                  }
                  frame #2 {
                    w5183 = "END"
                    n2792 = local read "mail control"() -> (w5184:string)
                    n2793 = case shown="False" w5179 {
                      tunnel: w5184 -> [w5208 _]
                      tunnel: w5183 -> [w5207 _]
                      tunnel: [w5206 FALSE] -> w5169
                      frame False {
                        n2794 = Equal?(x=w5208, y=w5207) -> (x = y?=w5206:bool)
                      }
                      frame True {
                      }
                    }
                    n2795 = case shown="False" w5185 {
                      tunnel: w5184 -> [w5224 _]
                      tunnel: w5183 -> [w5223 _]
                      tunnel: [w5222 FALSE] -> w5173
                      frame False {
                        n2796 = Equal?(x=w5224, y=w5223) -> (x = y?=w5222:bool)
                      }
                      frame True {
                      }
                    }
                    n2797 = case shown="False" w5182 {
                      tunnel: w5184 -> [w5220 _]
                      tunnel: w5183 -> [w5219 _]
                      tunnel: [w5218 FALSE] -> w5172
                      frame False {
                        n2798 = Equal?(x=w5220, y=w5219) -> (x = y?=w5218:bool)
                      }
                      frame True {
                      }
                    }
                    n2799 = case shown="False" w5180 {
                      tunnel: w5184 -> [w5212 _]
                      tunnel: w5183 -> [w5211 _]
                      tunnel: [w5210 FALSE] -> w5170
                      frame False {
                        n2800 = Equal?(x=w5212, y=w5211) -> (x = y?=w5210:bool)
                      }
                      frame True {
                      }
                    }
                    n2801 = case shown="False" w5181 {
                      tunnel: w5184 -> [w5216 _]
                      tunnel: w5183 -> [w5215 _]
                      tunnel: [w5214 FALSE] -> w5171
                      frame False {
                        n2802 = Equal?(x=w5216, y=w5215) -> (x = y?=w5214:bool)
                      }
                      frame True {
                      }
                    }
                    n2803 = Or(x=w5171, y=w5170) -> (x .or. y?=w5162:bool)
                    n2804 = Or(x=w5173, y=w5172) -> (x .or. y?=w5163:bool)
                    n2805 = Or(x=w5163, y=w5162) -> (x .or. y?=w5158:bool)
                    n2806 = case shown="False" w5175 {
                      tunnel: w5184 -> [w5192 _]
                      tunnel: w5183 -> [w5191 _]
                      tunnel: [w5190 FALSE] -> w5164
                      frame False {
                        n2807 = Equal?(x=w5192, y=w5191) -> (x = y?=w5190:bool)
                      }
                      frame True {
                      }
                    }
                    n2808 = case shown="False" w5174 {
                      tunnel: w5184 -> [w5188 _]
                      tunnel: w5183 -> [w5187 _]
                      tunnel: [w5186 FALSE] -> w5168
                      frame False {
                        n2809 = Equal?(x=w5188, y=w5187) -> (x = y?=w5186:bool)
                      }
                      frame True {
                      }
                    }
                    n2810 = case shown="False" w5176 {
                      tunnel: w5184 -> [w5196 _]
                      tunnel: w5183 -> [w5195 _]
                      tunnel: [w5194 FALSE] -> w5165
                      frame False {
                        n2811 = Equal?(x=w5196, y=w5195) -> (x = y?=w5194:bool)
                      }
                      frame True {
                      }
                    }
                    n2812 = case shown="False" w5178 {
                      tunnel: w5184 -> [w5204 _]
                      tunnel: w5183 -> [w5203 _]
                      tunnel: [w5202 FALSE] -> w5167
                      frame False {
                        n2813 = Equal?(x=w5204, y=w5203) -> (x = y?=w5202:bool)
                      }
                      frame True {
                      }
                    }
                    n2814 = case shown="False" w5177 {
                      tunnel: w5184 -> [w5200 _]
                      tunnel: w5183 -> [w5199 _]
                      tunnel: [w5198 FALSE] -> w5166
                      frame False {
                        n2815 = Equal?(x=w5200, y=w5199) -> (x = y?=w5198:bool)
                      }
                      frame True {
                      }
                    }
                    n2816 = Or(x=w5167, y=w5166) -> (x .or. y?=w5161:bool)
                    n2817 = Or(x=w5165, y=w5164) -> (x .or. y?=w5160:bool)
                    n2818 = Or(x=w5168, y=w5169) -> (x .or. y?=w5156:bool)
                    n2819 = Or(x=w5161, y=w5160) -> (x .or. y?=w5159:bool)
                    n2820 = Or(x=w5158, y=w5159) -> (x .or. y?=w5157:bool)
                    n2821 = Or(x=w5157, y=w5156) -> (x .or. y?=w5155:bool)
                  }
                  frame #3 {
                    n2822 = local read "on loops"() -> (w5238:dbl)
                    n2823 = local read "jig cycle"() -> (w5235:dbl)
                    n2824 = local read "Send Mail Now"() -> (w5229:bool)
                    n2825 = Add(x=w5238, y=3.0) -> (x+y=w5236:dbl)
                    n2826 = Equal?(x=w5235, y=w5236) -> (x = y?=w5230:bool)
                    n2827 = And(x=w5230, y=w5229) -> (x .and. y?=w5228:bool)
                    n2828 = And(x=w5234, y=w5230) -> (x .and. y?=w5233:bool)
                    n2829 = And(x=w5233, y=w5232) -> (x .and. y?=w5231:bool)
                    n2830 = Or(x=w5231, y=w5228) -> (x .or. y?=w5227:bool)
                    n2831 = case shown="True" w5227 {
                      tunnel: w5243 -> [_ w5249]
                      tunnel: w5242 -> [_ w5248]
                      tunnel: "Lab Panel Test Status" -> [_ w5247]
                      tunnel: w5240 -> [_ w5246]
                      tunnel: w5239 -> [_ w5245]
                      tunnel: w5226 -> [_ w5244]
                      frame False {
                      }
                      frame True {
                        n2832 = stacked-sequence {
                          tunnel: w5249 -> [w5257 _]
                          tunnel: w5248 -> [w5256 _]
                          tunnel: w5247 -> [w5255 _]
                          tunnel: w5246 -> [w5254 _]
                          tunnel: w5245 -> [w5253 _]
                          tunnel: w5244 -> [w5252 _]
                          frame #0 {
                            n2833 = call "sub vi - send mail v5.vi"("TO:"=w5257, "subject"=w5255, "from"=w5253, "out going server"=w5254, "message"=w5256) -> ("error out"=w5251:errorcluster)  [unwired: 10 in]
                            n2834 = Bundle(cluster=w5252, "mail error"=w5251) -> (w5250:T7)  [unwired: 6 in]
                            n2835 = local write "MAIL SETTINGS"(w5250) -> ()
                          }
                          frame #1 {
                            n2836 = local write "mail control"("") -> ()
                            n2837 = local write "Send Mail Now"(FALSE) -> ()
                          }
                        }
                      }
                    }
                  }
                }
              }
            }
          }
          frame #18 {
            # "save jig cycle values once all run switches are off"
            n2838 = stacked-sequence {
              tunnel: w5269 -> [_ w5298]
              tunnel: w5268 -> [_ w5297]
              tunnel: w5267 -> [_ w5296]
              tunnel: w5266 -> [_ w5295]
              tunnel: w5265 -> [_ w5294]
              tunnel: w5264 -> [_ w5293]
              tunnel: w5263 -> [_ w5292]
              tunnel: w5262 -> [_ w5291]
              tunnel: w5261 -> [_ w5290]
              tunnel: w5260 -> [_ w5289]
              frame #0 {
              }
              frame #1 {
                n2839 = Not(x=w5289) -> (.not. x?=w5272:bool)
                n2840 = Not(x=w5297) -> (.not. x?=w5287:bool)
                n2841 = Not(x=w5294) -> (.not. x?=w5282:bool)
                n2842 = Not(x=w5292) -> (.not. x?=w5278:bool)
                n2843 = Not(x=w5290) -> (.not. x?=w5274:bool)
                n2844 = Not(x=w5298) -> (.not. x?=w5288:bool)
                n2845 = Not(x=w5296) -> (.not. x?=w5286:bool)
                n2846 = Not(x=w5293) -> (.not. x?=w5280:bool)
                n2847 = Not(x=w5295) -> (.not. x?=w5284:bool)
                n2848 = Not(x=w5291) -> (.not. x?=w5276:bool)
                n2849 = local read "Save JC"() -> (w5300:bool)
                n2850 = And(x=w5288, y=w5287) -> (x .and. y?=w5285:bool)
                n2851 = And(x=w5285, y=w5286) -> (x .and. y?=w5283:bool)
                n2852 = And(x=w5283, y=w5284) -> (x .and. y?=w5281:bool)
                n2853 = And(x=w5281, y=w5282) -> (x .and. y?=w5279:bool)
                n2854 = And(x=w5279, y=w5280) -> (x .and. y?=w5277:bool)
                n2855 = And(x=w5277, y=w5278) -> (x .and. y?=w5275:bool)
                n2856 = And(x=w5275, y=w5276) -> (x .and. y?=w5273:bool)
                n2857 = And(x=w5273, y=w5274) -> (x .and. y?=w5271:bool)
                n2858 = And(x=w5271, y=w5272) -> (x .and. y?=w5270:bool)
                n2859 = And(x=w5270, y=w5300) -> (x .and. y?=w5299:bool)
                n2860 = case shown="True" w5299 {
                  tunnel: w5270 -> [w5301 _]
                  frame False {
                    n2861 = case shown="False" w5301 {
                      frame False {
                        n2862 = local write "Save JC"(TRUE) -> ()
                      }
                      frame True {
                      }
                    }
                  }
                  frame True {
                    n2863 = stacked-sequence {
                      frame #0 {
                        n2864 = String To Path(string="c:\\crabtree\\Jig Cycles\\") -> (path=w5313:path)
                        n2865 = Build Path(base path=w5313, name or relative path="jigcycles.bin") -> (appended path=w5311:path)
                        n2866 = Create Folder(path (use dialog)=w5313) -> (error out=w5315:errorcluster)  [unwired: 2 in, 2 out]
                        n2867 = local read "JIG RELAY CYCLES"() -> (w5305:T8)
                        n2868 = call <vilib>:"Clear Errors.vi"("error in (no error)"=w5315) -> ()  [unwired: 6 in, 1 out]
                        n2869 = local write "Save JC"(FALSE) -> ()
                        n2870 = Open/Create/Replace File(file path (use dialog)=w5311, operation (0:open)=T21."replace or create") -> (refnum out=w5309:refnum<file>, error out=w5310:errorcluster)  [unwired: 4 in, 1 out]
                        n2871 = Write to Binary File(file (use dialog)=w5309, data=w5305, error in=w5310) -> (refnum out=w5308:refnum<file>, error out=w5307:errorcluster)  [unwired: 3 in, 1 out]
                        n2872 = Close File(refnum=w5308, error in=w5307) -> (error out=w5306:errorcluster)  [unwired: 1 out]
                        n2873 = local write "data file error"(w5306) -> ()
                      }
                      frame #1 {
                        n2874 = local read "JIG RELAY CYCLES"() -> (w5338:T8)
                        n2875 = Unbundle By Name(w5338) -> ("LAB01-1"=w5333:dbl, "LAB01-2"=w5332:dbl, "LAB02-1"=w5330:dbl, "LAB02-2"=w5329:dbl, "LAB03-1"=w5327:dbl, "LAB03-2"=w5324:dbl, "LAB04-1"=w5323:dbl, "LAB04-2"=w5321:dbl, "LAB05-1"=w5319:dbl, "LAB05-2"=w5317:dbl)
                        n2876 = stacked-sequence {
                          tunnel: w5333 -> [w5341 _ _ _ _ _ _ _ _ _]
                          tunnel: 1000000 -> [w5344 w5354 w5364 w5374 w5384 w5394 w5404 w5414 w5424 w5434]
                          tunnel: [w5342 _ _ _ _ _ _ _ _ _] -> w5336
                          tunnel: "TEST STATION HAS REACHED 1 MILLION CYCLES, REPLACE  CONTROL RELAYS" -> [w5340 w5352 w5362 w5372 w5382 w5392 w5402 w5412 w5422 w5432]
                          tunnel: [_ w5351 _ _ _ _ _ _ _ _] -> w5334
                          tunnel: w5332 -> [_ w5350 _ _ _ _ _ _ _ _]
                          tunnel: [_ _ w5361 _ _ _ _ _ _ _] -> w5331
                          tunnel: w5330 -> [_ _ w5360 _ _ _ _ _ _ _]
                          tunnel: w5329 -> [_ _ _ w5371 _ _ _ _ _ _]
                          tunnel: [_ _ _ w5370 _ _ _ _ _ _] -> w5328
                          tunnel: w5327 -> [_ _ _ _ w5381 _ _ _ _ _]
                          tunnel: [_ _ _ _ w5380 _ _ _ _ _] -> w5326
                          tunnel: [_ _ _ _ _ w5391 _ _ _ _] -> w5325
                          tunnel: w5324 -> [_ _ _ _ _ w5390 _ _ _ _]
                          tunnel: w5323 -> [_ _ _ _ _ _ w5401 _ _ _]
                          tunnel: [_ _ _ _ _ _ w5400 _ _ _] -> w5322
                          tunnel: w5321 -> [_ _ _ _ _ _ _ w5411 _ _]
                          tunnel: [_ _ _ _ _ _ _ w5410 _ _] -> w5320
                          tunnel: w5319 -> [_ _ _ _ _ _ _ _ w5421 _]
                          tunnel: [_ _ _ _ _ _ _ _ w5420 _] -> w5318
                          tunnel: w5317 -> [_ _ _ _ _ _ _ _ _ w5431]
                          tunnel: [_ _ _ _ _ _ _ _ _ w5430] -> w5316
                          frame #0 {
                            n2877 = Greater?(x=w5341, y=w5344) -> (0:w5343:bool)
                            n2878 = case shown="True" w5343 {
                              tunnel: [w5345 0] -> w5342
                              tunnel: w5341 -> [w5345 _]
                              tunnel: w5340 -> [_ w5346]
                              frame False {
                              }
                              frame True {
                                n2879 = Concatenate Strings("LA01-1 ", w5346) -> (w5349:string)
                                n2880 = One Button Dialog(message=w5349) -> ()  [unwired: 1 in, 1 out]
                              }
                            }
                          }
                          frame #1 {
                            n2881 = Greater?(x=w5350, y=w5354) -> (0:w5353:bool)
                            n2882 = case shown="True" w5353 {
                              tunnel: [w5355 0] -> w5351
                              tunnel: w5350 -> [w5355 _]
                              tunnel: w5352 -> [_ w5356]
                              frame False {
                              }
                              frame True {
                                n2883 = Concatenate Strings("LA01-2 ", w5356) -> (w5359:string)
                                n2884 = One Button Dialog(message=w5359) -> ()  [unwired: 1 in, 1 out]
                              }
                            }
                          }
                          frame #2 {
                            n2885 = Greater?(x=w5360, y=w5364) -> (0:w5363:bool)
                            n2886 = case shown="True" w5363 {
                              tunnel: [w5365 0] -> w5361
                              tunnel: w5360 -> [w5365 _]
                              tunnel: w5362 -> [_ w5366]
                              frame False {
                              }
                              frame True {
                                n2887 = Concatenate Strings("LA02-1 ", w5366) -> (w5369:string)
                                n2888 = One Button Dialog(message=w5369) -> ()  [unwired: 1 in, 1 out]
                              }
                            }
                          }
                          frame #3 {
                            n2889 = Greater?(x=w5371, y=w5374) -> (0:w5373:bool)
                            n2890 = case shown="True" w5373 {
